vi "SetRefSearchParameters.vi"(0 "handle in":i32, 1 "UnitAddress(0)":u16, 2 "MotNr(0)":u8, 5 "error in":errorcluster, 7 "Ref Search Parameter":T1={"VRefMax(100)"=100, "DebouncingTime (22ms)"=34} {"DebouncingTime (22ms)" format="%.0x"}) -> (14 "handle out":i32, 19 "error out":errorcluster)   [LabVIEW 2014, in "Sixpack - Driver.lvlib"]
doc: "ACHTUNG: VRefMax gilt nur für die schnelle Referenzfahrtrelevant. nur bei stehendem Motor ändern!\n\nDie Variable DebouncingTime gibt direkt die Zeit an (maximal 30, nur gerade Zahlen erlaubt). Mask (P3/P4) wird dann automatisch erzeugt.\n\nCMD $16\nMotorNr (0...5)\nVRefMax (1..511): Referenzfahrt- Maximalgeschwindigkeit\n VMax >= VRefMax >= VStart; VRefMax <= 511\nDebouncingTime:\n Maske für Referenzschalterentprellung ($0001=0ms, $0003=2ms, ...$FFFF=30ms) \n Default = $0FFF (=22ms)\nSTOPAFTERREF\n 0 = macht nach Referenzfahrt mit akt. Aktion weiter\n 1 = Stopp nach Referenzfahrt"
uses:
  Sixpack - Driver.lvlib
  Ref Search Parameter.ctl
  DLL/PackDLL.dll
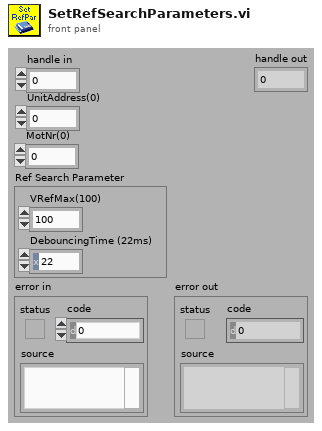
[diagram p1: front panel]
types:
  T1 = typedef "Sixpack - Driver.lvlib/Ref Search Parameter.ctl" = cluster{"VRefMax(100)":u16, "DebouncingTime (22ms)":u8}
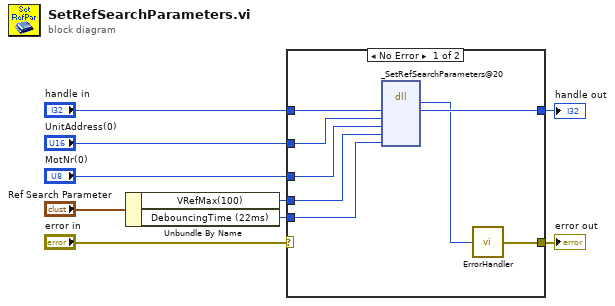
[diagram p0: block diagram]
diagram:
  n1 = Unbundle By Name("Ref Search Parameter") -> ("VRefMax(100)"=w2:u16, "DebouncingTime (22ms)"=w1:u8)
  n2 = case shown="No Error" "error in" {
    selector: "error in" -> [_ w19]
    tunnel: "handle in" -> [w17 w18]
    tunnel: [w16 w18] -> w8
    tunnel: "UnitAddress(0)" -> [w15 _]
    tunnel: "MotNr(0)" -> [w14 _]
    tunnel: w2 -> [w13 _]
    tunnel: w1 -> [w12 _]
    tunnel: [w11 w19] -> w4
    frame No Error {
      n3 = dll-call lib="D:/CS-Source/LV2014/GPL/instr.lib/SixPack/PackDLL/DLL/PackDLL.dll" fn="_SetRefSearchParameters@20" label="SetRefSearchParameters"("HANDLE"=w17, "UnitAddress"=w15, "MotNr"=w14, "VRefMax"=w13, "DebouncingTime"=w12) -> ("BOOLEAN"=w10:i8, "HANDLE"=w16:i32)  [unwired: 7 in, 2 out]
      n4 = call "ErrorHandler.vi"("BOOLEAN"=w10) -> ("error out"=w11:errorcluster)
    }
    frame Error {
    }
  }
  "handle out" <- w8
  "error out" <- w4
